vi "Write lastUpdateTime.vi"(8 "error in (no error)":errorcluster, 10 "lastUpdateTime":dbl, 11 "deviceHeartbeat in":refnum<class "deviceHeartbeat.lvclass">) -> (0 "error out":errorcluster, 3 "deviceHeartbeat out":refnum<class "deviceHeartbeat.lvclass">)   [LabVIEW 2016, in "deviceHeartbeat.lvclass"]
uses:
  deviceHeartbeat.lvclass
  deviceHeartbeat.lvclass/deviceHeartbeat.ctl
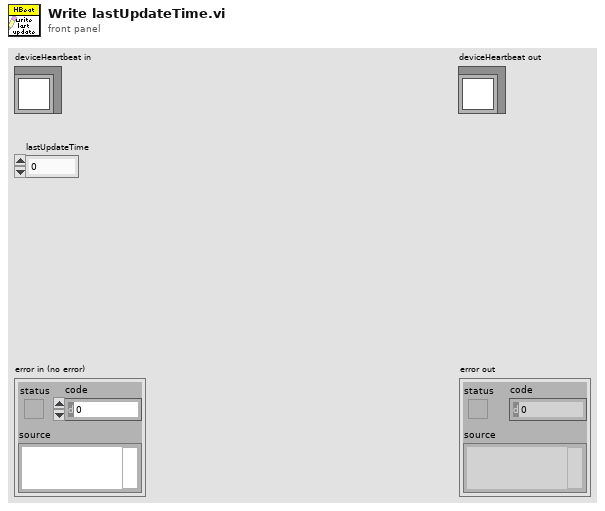
[diagram p1: front panel]
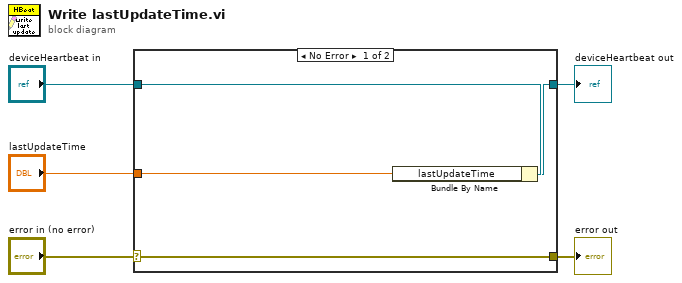
[diagram p0: block diagram]
diagram:
  n1 = case shown="No Error" "error in (no error)" {
    selector: "error in (no error)" -> [w9 w10]
    tunnel: [w9 w10] -> w4
    tunnel: [w7 w11] -> w2
    tunnel: "deviceHeartbeat in" -> [w8 w11]
    tunnel: "lastUpdateTime" -> [w6 _]
    frame No Error {
      n2 = Bundle By Name(cluster=w8, "lastUpdateTime"=w6) -> (w7:refnum<class "deviceHeartbeat.lvclass">)
    }
    frame Error {
    }
  }
  "error out" <- w4
  "deviceHeartbeat out" <- w2
